vi "Init Control.vi"(5 "Group":refnum<class "Group DBL.lvclass">, 6 "Period ms":i64, 7 "VolatusAPI":refnum<class "VolatusAPI.lvclass">, 8 "error in (no error)":errorcluster, 9 "Control MsgQ":refnum<class "MessageQ.lvclass">, 10 "Config Element":refnum<class "Config Element.lvclass">, 11 "Valve in":refnum<class "HitAndHoldControl.lvclass">) -> (0 "error out":errorcluster, 3 "Valve out":refnum<class "HitAndHoldControl.lvclass">)   [LabVIEW 2020, in "VolatusControl.lvlib" / "HitAndHoldControl.lvclass"]
uses:
  HitAndHoldControl.lvclass
  HitAndHoldControl.lvclass/HitAndHoldControl.ctl
  lv-cdm/CDM-Config/Config Element/Config Element.lvclass
  VolatusControl.lvlib
  lv-vecto/Vecto/Group/Group.lvclass
  Volatus/VolatusAPI/VolatusAPI.lvclass
  lv-vecto/Vecto/Group DBL/Group DBL.lvclass
  C:/dev/lv20CE/relink/lv-vecto/Vecto/Group/Group.lvclass
  C:/dev/lv20CE/relink/lv-vecto/Vecto/Group DBL/Group DBL.lvclass
  Volatus/MessageQ/MessageQ.lvclass
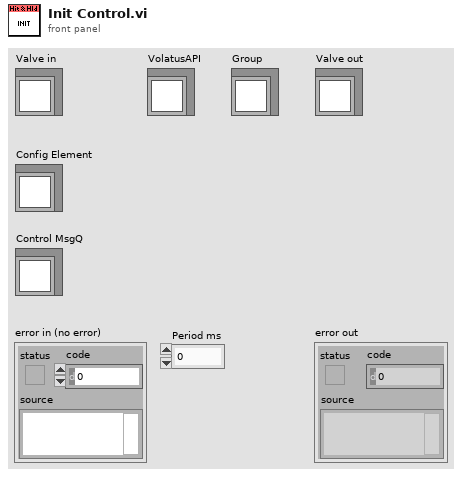
[diagram p1: front panel]
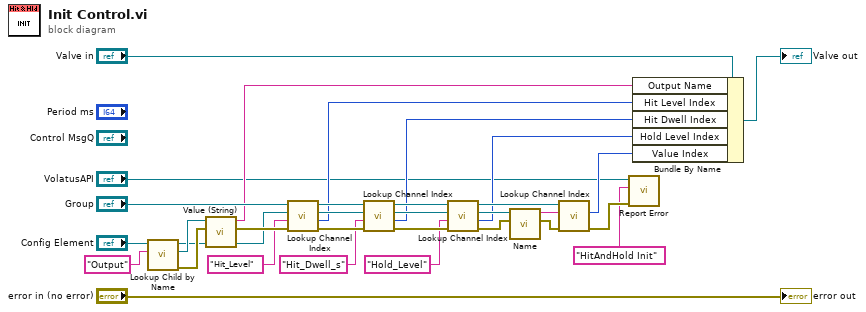
[diagram p0: block diagram]
diagram:
  n1 = call "Lookup Child by Name.vi"("Name"="Output", "Config Element in"="Config Element") -> ("error out"=w25:errorcluster, "Child"=w26:refnum<class "Config Element.lvclass">, "Config Element out"=w19:refnum<class "Config Element.lvclass">)  [unwired: 6 in, 1 out]
  n2 = call "Value (String).vi"("error in (no error)"=w25, "Config Element in"=w26) -> ("error out"=w23:errorcluster, "String Value"=w21:string)  [unwired: 8 in]
  n3 = call "Lookup Channel Index.vi"("error in (no error)"=w23, "Meta Value"="Hit_Level" ("Name"), "Config Element in"=w19, "Group in"="Group") -> ("error out"=w16:errorcluster, "Index"=w4:i32, "Config Element"=w17:refnum<class "Config Element.lvclass">, "Group"=w18:refnum<class "Group DBL.lvclass">)  [unwired: 4 in]
  n4 = call "Lookup Channel Index.vi"("error in (no error)"=w16, "Meta Value"="Hit_Dwell_s" ("Name"), "Config Element in"=w17, "Group in"=w18) -> ("error out"=w31:errorcluster, "Index"=w5:i32, "Config Element"=w12:refnum<class "Config Element.lvclass">, "Group"=w13:refnum<class "Group DBL.lvclass">)  [unwired: 4 in]
  n5 = call "Lookup Channel Index.vi"("error in (no error)"=w31, "Meta Value"="Hold_Level" ("Name"), "Config Element in"=w12, "Group in"=w13) -> ("error out"=w7:errorcluster, "Index"=w6:i32, "Config Element"=w11:refnum<class "Config Element.lvclass">, "Group"=w10:refnum<class "Group DBL.lvclass">)  [unwired: 4 in]
  n6 = call "Name.vi"("error in (no error)"=w7, "Config Element in"=w11) -> ("error out"=w8:errorcluster, "Name"=w9:string)  [unwired: 8 in]
  n7 = call "Lookup Channel Index.vi"("error in (no error)"=w8, "Channel Name"=w9, "Group in"=w10) -> ("error out"=w32:errorcluster, "Index"=w3:i32)  [unwired: 6 in, 1 out]
  n8 = call "Report Error.vi"("error in (no error)"=w32, "Context"="HitAndHold Init", "VolatusAPI in"="VolatusAPI") -> ()  [unwired: 7 in, 2 out]
  n9 = Bundle By Name(cluster="Valve in", "Output Name"=w21, "Hit Level Index"=w4, "Hit Dwell Index"=w5, "Hold Level Index"=w6, "Value Index"=w3) -> (→"Valve out":refnum<class "HitAndHoldControl.lvclass">)
  "error out" <- "error in (no error)"
